vi "Load Help File.vi"(8 "error in (no error)":errorcluster, 9 "HTML File to Load":string, 11 "Browser":refnum<k7>(container)) -> (0 "error out":errorcluster)   [LabVIEW 2020, in "Communication Bus Template System Explorer.lvlib" / "Implementation.lvlib"]
doc: "Loads the specified HTML page from the CHM into the browser"
uses:
  Implementation.lvlib
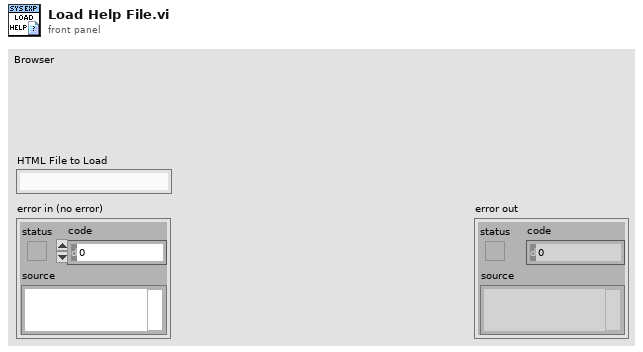
[diagram p1: front panel]
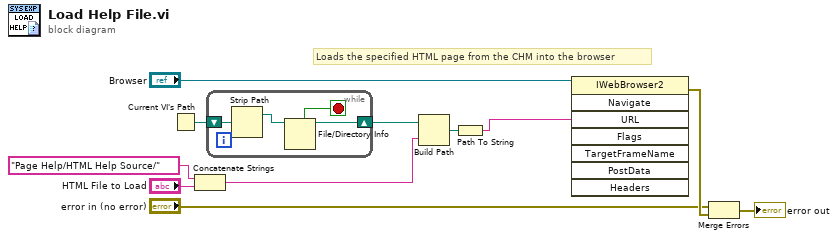
[diagram p0: block diagram]
diagram:
  # "Loads the specified HTML page from the CHM into the browser"
  n1 = Current VI's Path() -> (path=w11:path)
  n2 = Concatenate Strings("Page Help/HTML Help Source/", "HTML File to Load") -> (w2:string)
  n3 = while {
    shift-right: [w13] -> w5
    shift-left: w11 -> [w15]
    stop <- w12 stop-if-true
    n4 = Strip Path(path=w15) -> (stripped path=w14:path)  [unwired: 1 out]
    n5 = File/Directory Info(path=w14) -> (path out=w13:path, directory=w12:bool)  [unwired: 1 in, 5 out]
  }
  n6 = Build Path(base path=w5, name or relative path=w2) -> (appended path=w10:path)
  n7 = Path To String(path=w10) -> (string=w3:string)
  n8 = invoke class="IWebBrowser2" method="Navigate"(reference="Browser", "URL"=w3) -> (error out=w8:errorcluster)  [unwired: 6 in, 7 out]
  n9 = Merge Errors("error in (no error)", w8) -> (→"error out":errorcluster)
